vi "Tetra_TX-PROD_Close.vi"() -> (0 "error out":errorcluster, 2 "Status":string)   [LabVIEW 2018]
uses:
  Infrastructure/Test Parameter Globals_1.0.0.vi
  Initialize References/Station References Global.vi
  Tetra_Globals.vi
  Instruments/PNA/lib functions/Agilent ENA Series.lvlib
panel:
  in  "Close ComPort(t)":bool=TRUE
  in  "Close Oven(t)":bool=TRUE
  out "Use PS1-2":bool=TRUE
  out "PS1-2(A)":dbl=1.0
  out "PS1-2(V)":dbl=5.0
  out "Use PS1-1":bool=TRUE
  out "Text":refnum<vi>
  in  "Close  PNA (T)":bool=TRUE
  in  "Close Power Supply (T)":bool=TRUE
  in  "error in (no error)":errorcluster
  out "PS1-1(A)":dbl=1.0
  out "PS1-1(V)":dbl=18.75
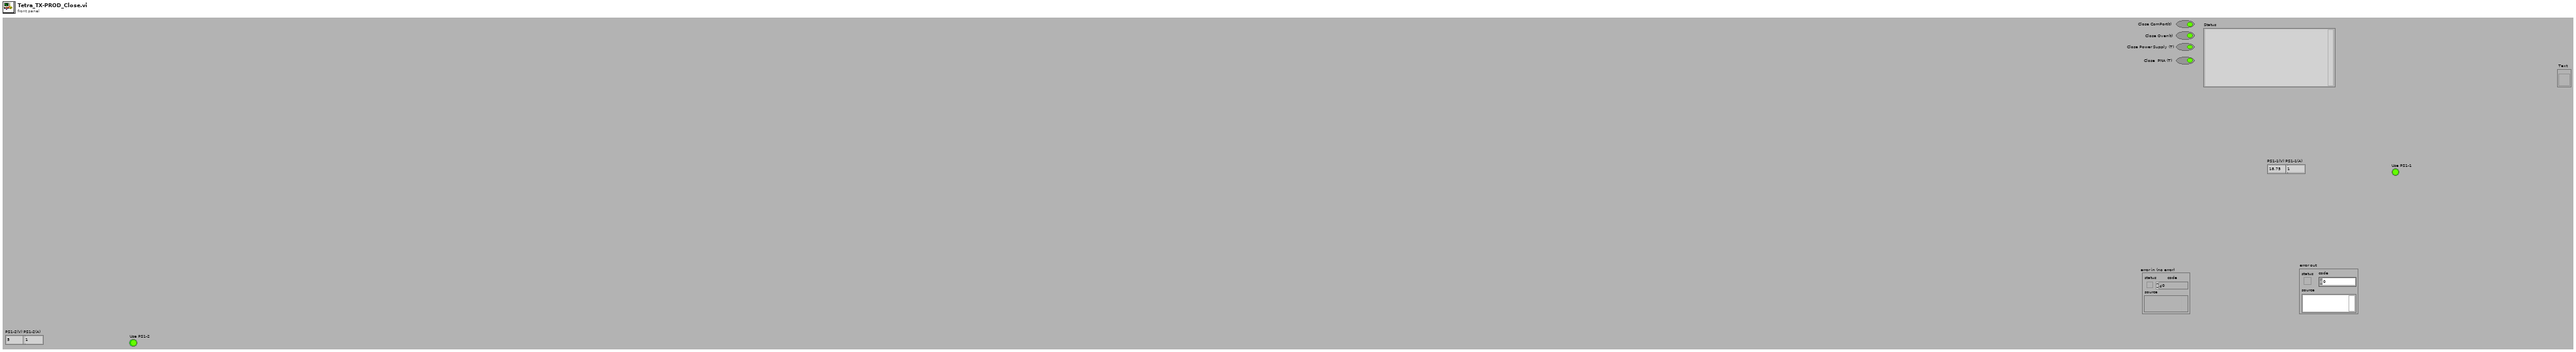
[diagram p1: front panel]
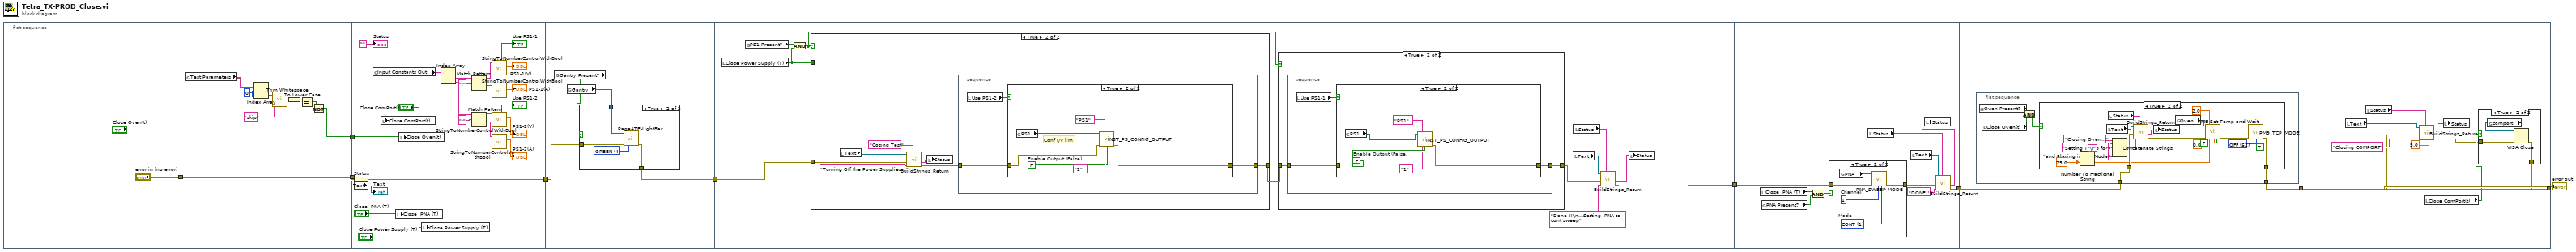
[diagram p0: block diagram]
diagram:
  n1 = flat-sequence {
    tunnel: ["error in (no error)"] -> w5
    tunnel: w5 -> [w19]
    tunnel: [w19] -> w4
    tunnel: [w11] -> w1
    tunnel: [w32] -> w3
    tunnel: w4 -> [w22]
    tunnel: w1 -> [w20]
    tunnel: w3 -> [w44]
    tunnel: [w43] -> w2
    tunnel: [w55] -> w6
    tunnel: w2 -> [w62]
    tunnel: [w101] -> w8
    tunnel: w6 -> [w97]
    tunnel: w8 -> [w109]
    tunnel: [w110] -> w7
    tunnel: [w138] -> w9
    tunnel: w7 -> [w141]
    frame #0 {
    }
    frame #1 {
      w17 = 0 ("index (row)")
      n2 = global read "Test Parameter Globals_1.0.0.vi" "Test Parameters"() -> (w18:string[][])
      n3 = Index Array(array=w18, index (row)=w17, index (col)=w17) -> (element=w16:string)
      n4 = call <vilib>:"Trim Whitespace.vi"("string"=w16) -> ("trimmed string"=w14:string)  [unwired: 1 in]
      n5 = To Lower Case(string=w14) -> (all lower case string=w13:string)
      n6 = Equal?(x=w13, y="skip") -> (x = y?=w12:bool)
      n7 = Not(x=w12) -> (.not. x?=w11:bool)
    }
    frame #2 {
      n8 = property on="Status" class="Str"(error in=w22) -> (error out=w32:errorcluster, "Text"=→"Text":refnum<vi>)  [unwired: 1 in, 1 out]
      n9 = global read "Test Parameter Globals_1.0.0.vi" "Input Constants Out"() -> (w23:string[])
      n10 = local write "Close ComPort(t)"("Close ComPort(t)") -> ()
      n11 = local write "Close  PNA (T)"("Close  PNA (T)") -> ()
      n12 = local write "Close Oven(t)"(w20) -> ()
      n13 = local write "Close Power Supply (T)"("Close Power Supply (T)") -> ()
      n14 = Index Array(array=w23) -> (element #1=w31:string, element #2=w24:string)  [unwired: 2 in]
      n15 = Match Pattern(string=w31, regular expression=";") -> (before substring=w37:string, after substring=w36:string)  [unwired: 1 in, 2 out]
      n16 = Match Pattern(string=w24, regular expression=";") -> (before substring=w29:string, after substring=w28:string)  [unwired: 1 in, 2 out]
      n17 = call "StringToNumberControlWithBool.vi"("String In"=w37) -> ("Number Out"=→"PS1-1(V)":dbl, "NOT = 0"=→"Use PS1-1":bool)  [unwired: 7 in]
      n18 = call "StringToNumberControlWithBool.vi"("String In"=w36) -> ("Number Out"=→"PS1-1(A)":dbl)  [unwired: 7 in, 1 out]
      n19 = call "StringToNumberControlWithBool.vi"("String In"=w29) -> ("Number Out"=→"PS1-2(V)":dbl, "NOT = 0"=→"Use PS1-2":bool)  [unwired: 7 in]
      n20 = call "StringToNumberControlWithBool.vi"("String In"=w28) -> ("Number Out"=→"PS1-2(A)":dbl)  [unwired: 7 in, 1 out]
      "Status" <- ""
    }
    frame #3 {
      n21 = global read "Station References Global.vi" "Gantry Present?"() -> (w46:bool)
      n22 = global read "Station References Global.vi" "Gantry"() -> (w45:refnum<visa-resource-name>)
      n23 = case shown="True" w46 {
        tunnel: w45 -> [_ w51]
        tunnel: w44 -> [w47 w50]
        tunnel: [w47 w49] -> w43
        frame False {
        }
        frame True {
          w48 = u32 4 items=["OFF"=0, "RED"=1, "AMBER"=2, "GREEN"=4, "ALL"=7, "BUZZ"=8, "RED+BUZZ"=9, "ALL+BUZZ"=15] ("Select")
          n24 = call "RageATE-LightBar.vi"("VISA resource name"=w51, "error in"=w50, "Select"=w48) -> ("error out"=w49:errorcluster)  [unwired: 10 in, 2 out]
        }
      }
    }
    frame #4 {
      n25 = local read "Close Power Supply (T)"() -> (w56:bool)
      n26 = global read "Station References Global.vi" "PS1 Present?"() -> (w61:bool)
      n27 = And(x=w61, y=w56) -> (x .and. y?=w58:bool)
      n28 = case shown="True" w58 {
        tunnel: [w75 w78] -> w59
        tunnel: w62 -> [w75 w80]
        tunnel: w56 -> [_ _]
        frame False {
        }
        frame True {
          n29 = local read "Text"() -> (w76:refnum<vi>)
          n30 = call "BuildStrings_Return.vi"("Input String"="Cosing Test", "New String"="Turning Off the Power Supplies...", "error in (no error)"=w80, "reference"=w76) -> ("error out"=w79:errorcluster, "concatenated string"=w77:string)  [unwired: 5 in, 1 out]
          n31 = local write "Status"(w77) -> ()
          n32 = stacked-sequence {
            tunnel: w79 -> [w85]
            tunnel: [w83] -> w78
            frame #0 {
              n33 = local read "Use PS1-2"() -> (w84:bool)
              n34 = case shown="True" w84 {
                tunnel: [w86 w87] -> w83
                tunnel: w85 -> [w86 w91]
                frame False {
                }
                frame True {
                  w88 = FALSE  # Enable Output (False)
                  # "Conf I/V lim"
                  n35 = global read "Station References Global.vi" "PS1"() -> (w92:refnum<visa-resource-name>)
                  n36 = call "INST_PS_CONFIG_OUTPUT.vi"("VISA session"=w92, "SEL_PS"="PS1", "error in (no error)"=w91, "Instrument Select (Output 1)"="2", "Enable Output (False)"=w88) -> ("error out"=w87:errorcluster)  [unwired: 8 in, 2 out]
                }
              }
            }
          }
        }
      }
      n37 = case shown="True" w58 {
        tunnel: [w63 w65] -> w57
        tunnel: w59 -> [w63 w64]
        frame False {
        }
        frame True {
          n38 = stacked-sequence {
            tunnel: w64 -> [w68]
            tunnel: [w66] -> w65
            frame #0 {
              n39 = local read "Use PS1-1"() -> (w67:bool)
              n40 = case shown="True" w67 {
                tunnel: [w69 w70] -> w66
                tunnel: w68 -> [w69 _]
                frame False {
                }
                frame True {
                  w73 = FALSE  # Enable Output (False)
                  n41 = global read "Station References Global.vi" "PS1"() -> (w74:refnum<visa-resource-name>)
                  n42 = call "INST_PS_CONFIG_OUTPUT.vi"("VISA session"=w74, "SEL_PS"="PS1", "Instrument Select (Output 1)"="1", "Enable Output (False)"=w73) -> ("error out"=w70:errorcluster)  [unwired: 9 in, 2 out]
                }
              }
            }
          }
        }
      }
      n43 = local read "Text"() -> (w54:refnum<vi>)
      n44 = local read "Status"() -> (w53:string)
      n45 = call "BuildStrings_Return.vi"("Input String"=w53, "New String"="Done !!!\n...Setting  PNA to cont sweep", "error in (no error)"=w57, "reference"=w54) -> ("error out"=w55:errorcluster, "concatenated string"=w52:string)  [unwired: 5 in, 1 out]
      n46 = local write "Status"(w52) -> ()
    }
    frame #5 {
      n47 = local read "Close  PNA (T)"() -> (w100:bool)
      n48 = global read "Station References Global.vi" "PNA Present?"() -> (w99:bool)
      n49 = And(x=w100, y=w99) -> (x .and. y?=w98:bool)
      n50 = case shown="True" w98 {
        tunnel: w97 -> [w103 w106]
        tunnel: [w103 w104] -> w96
        frame False {
        }
        frame True {
          w107 = 1 items=["HOLD", "CONT", "GROUP", "SINGLE"]  # Mode
          w108 = 1  # Channel
          n51 = global read "Station References Global.vi" "PNA"() -> (w105:refnum<visa-resource-name>)
          n52 = call "PNA_SWEEP MODE.vi"("Mode"=w107, "Channel"=w108, "error in (no error)"=w106, "VISA resource name"=w105) -> ("error out"=w104:errorcluster)  [unwired: 6 in, 1 out]
        }
      }
      n53 = local read "Status"() -> (w94:string)
      n54 = local read "Text"() -> (w95:refnum<vi>)
      n55 = call "BuildStrings_Return.vi"("Input String"=w94, "New String"="DONE!!!", "error in (no error)"=w96, "reference"=w95) -> ("error out"=w101:errorcluster, "concatenated string"=w93:string)  [unwired: 5 in, 1 out]
      n56 = local write "Status"(w93) -> ()
    }
    frame #6 {
      n57 = flat-sequence {
        tunnel: [w115] -> w110
        tunnel: w109 -> [w114]
        frame #0 {
          n58 = global read "Station References Global.vi" "Oven Present?"() -> (w113:bool)
          n59 = local read "Close Oven(t)"() -> (w111:bool)
          n60 = And(x=w113, y=w111) -> (x .and. y?=w112:bool)
          n61 = case shown="True" w112 {
            tunnel: [w116 w137] -> w115
            tunnel: w114 -> [w116 w131]
            frame False {
            }
            frame True {
              w122 = 25.0 ("Set Point")
              w136 = u16 62 items=["READ ONLY"=0, "AUTO"=10, "OFF"=62, "MAN"=54] ("MODE")
              n62 = Number To Fractional String(number=w122) -> (F-format string=w121:string)  [unwired: 3 in]
              n63 = local read "Text"() -> (w133:refnum<vi>)
              n64 = local read "Status"() -> (w134:string)
              n65 = Concatenate Strings("Closing Oven..." ("New String"), "\r", "Setting Temp for " ("string"), w121, "and Placing in OFF Mode" ("string")) -> (w125:string)
              n66 = call "BuildStrings_Return.vi"("Input String"=w134, "New String"=w125, "error in (no error)"=w131, "reference"=w133) -> ("error out"=w126:errorcluster, "concatenated string"=w130:string)  [unwired: 5 in, 1 out]
              n67 = local write "Status"(w130) -> ()
              n68 = global read "Station References Global.vi" "Oven"() -> (w127:refnum<visa-resource-name>)
              n69 = call "PM9 Set Temp and Wait.vi"("VISA"=w127, "Error In"=w126, "Accuracy +/-"=2.0, "Set Point"=w122, "Min (-1 for cont.)"=0.0, "close session(t)"=FALSE) -> ("visa"=w128:refnum<visa-resource-name>, "error out"=w129:errorcluster)  [unwired: 10 in, 2 out]
              n70 = call "PM9_TCP_MODE.vi"("VISA"=w128, "error in (no error)"=w129, "MODE"=w136, "Close tcp(t)"=TRUE) -> ("error out"=w137:errorcluster)  [unwired: 8 in, 3 out]
            }
          }
        }
      }
    }
    frame #7 {
      n71 = local read "Text"() -> (w146:refnum<vi>)
      n72 = local read "Status"() -> (w145:string)
      n73 = call "BuildStrings_Return.vi"("seconds to wait"=5.0, "Input String"=w145, "New String"="Closing COMPORT", "error in (no error)"=w141, "reference"=w146) -> ("error out"=w139:errorcluster, "concatenated string"=w144:string)  [unwired: 4 in, 1 out]
      n74 = local read "Close ComPort(t)"() -> (w140:bool)
      n75 = local write "Status"(w144) -> ()
      n76 = case shown="True" w140 {
        tunnel: w139 -> [w147 w149]
        tunnel: [w147 w148] -> w138
        frame False {
        }
        frame True {
          n77 = global read "Tetra_Globals.vi" "comport"() -> (w150:refnum<visa-resource-name>)
          n78 = VISA Close(VISA resource name=w150, error in (no error)=w149) -> (error out=w148:errorcluster)
        }
      }
    }
  }
  "error out" <- w9
